vi "Action.vi"(8 "b":dbl, 10 "a":dbl, 11 "add in":refnum<class "subtract.lvclass">) -> (1 "result":dbl, 3 "add out":refnum<class "subtract.lvclass">)   [LabVIEW 2020, in "subtract.lvlib" / "subtract.lvclass"]
uses:
  subtract.lvclass
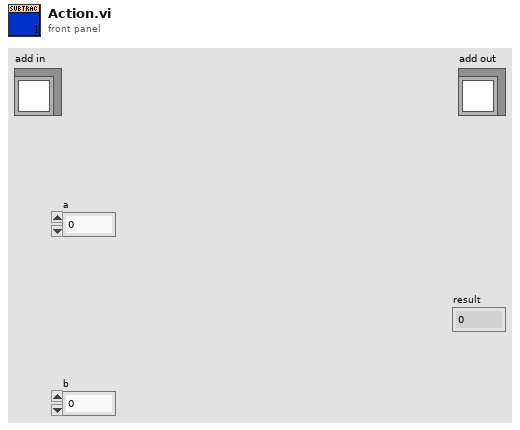
[diagram p1: front panel]
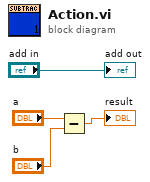
[diagram p0: block diagram]
diagram:
  n1 = Subtract(x="a", y="b") -> (x-y=→"result":dbl)
  "add out" <- "add in"
